vi "Number of files loaded.vi"(0 "APG Config":T1, 5 "IPF temp Folder":path, 11 "error in (no error)":errorcluster) -> (15 "error out":errorcluster)   [LabVIEW 2013, in "Manipulate IPF.lvlib"]
uses:
  Manipulate IPF.lvlib
  Settings/type_def/APG Config.ctl
  <userlib>/_OpenG.lib/file/file.llb/File Exists - Scalar__ogtk.vi
  <userlib>/_OpenG.lib/file/file.llb/Valid Path - Traditional__ogtk.vi
  a3Di APG.lvlib
  Settings/APG_settings.lvlib
panel:
  out "# of file loaded":string
  # "IPF Files Loaded"
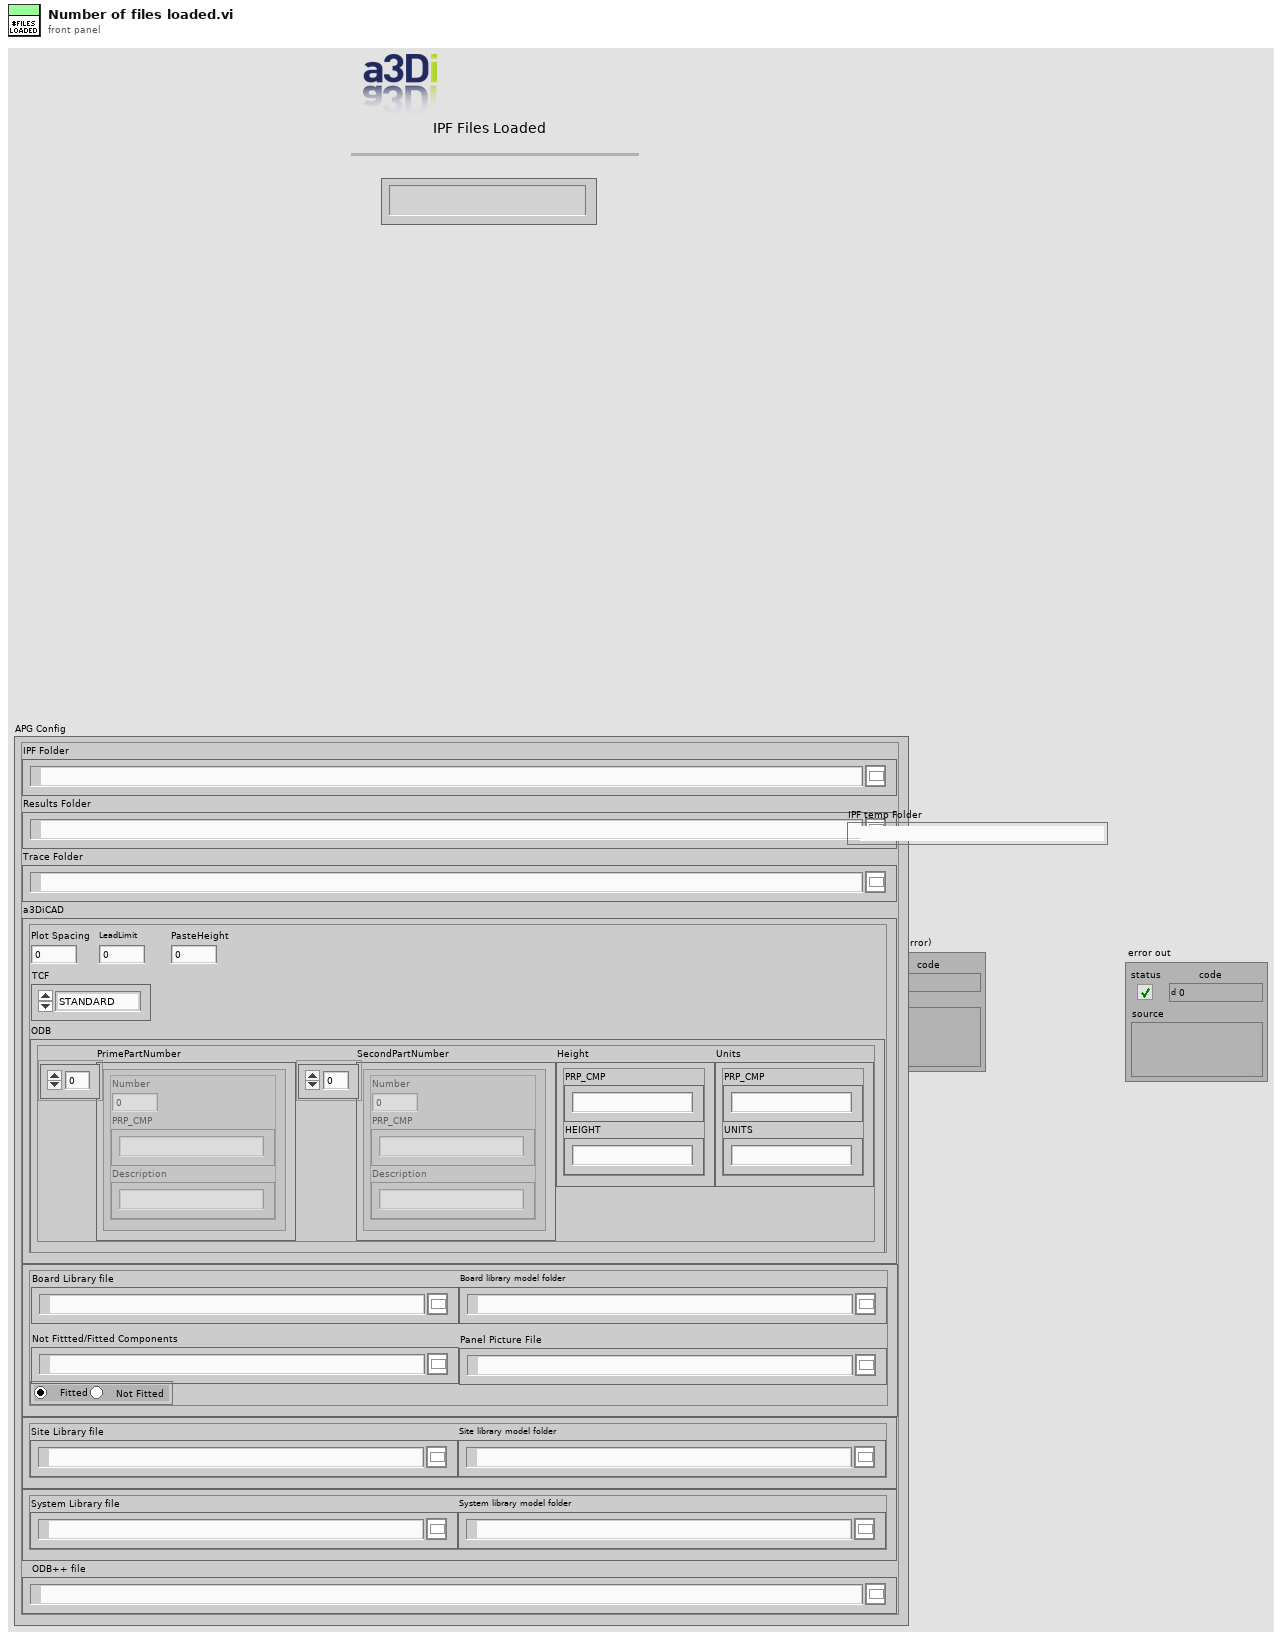
[diagram p1: front panel]
types:
  T1 = typedef "APG_settings.lvlib/APG Config.ctl" = cluster{"IPF Folder":path, "Results Folder":path, "Trace Folder":path, "a3DiCAD":cluster{"Plot Spacing":dbl, "TCF":enum16{"STANDARD", "PASTE", "LEAD"}, "LeadLimit":u32, "a3DiCADDebug":bool, "ODB":cluster{"PrimePartNumber":cluster{"Number":u32, "PRP_CMP":string, "Description":string}[], "SecondPartNumber":cluster{"Number":u32, "PRP_CMP":string, "Description":string}[], "Height":cluster{"PRP_CMP":string, "HEIGHT":string}, "Units":cluster{"PRP_CMP":string, "UNITS":string}}, "PasteHeight":dbl}, "a3DiCADcfg":path, "Board Library":cluster{"Board Library file":path, "Board library model folder":path, "Not Fittted/Fitted Components":path, "Panel Picture File":path, "Components":enum32{"Fitted", "Not Fitted "}}, "Site Library":cluster{"Site Library file":path, "Site library model folder":path}, "System Library":cluster{"System Library file":path, "System library model folder":path}, "ODB++ file":path}
  T2 = enum32{"Invalid", "Standard", "Closed", "Hidden", "Minimized", "Maximized"}
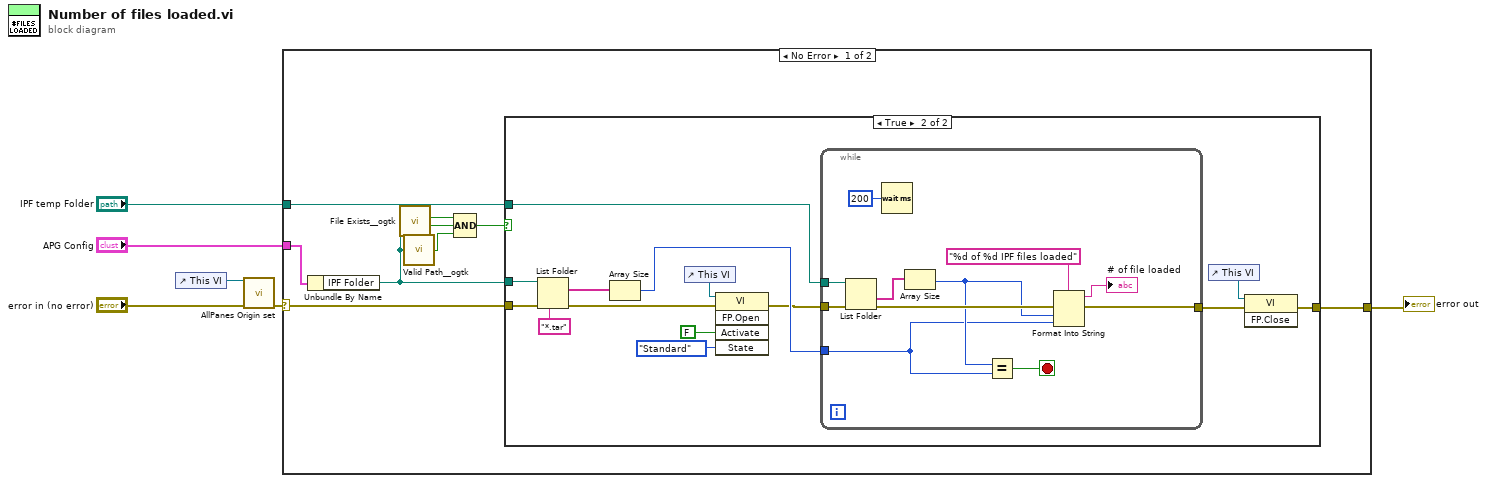
[diagram p0: block diagram]
diagram:
  n1 = control-ref of="This VI"() -> (w6:refnum<vi>)
  n2 = call "AllPanes Origin set.vi"("VI ref in"=w6, "error in"="error in (no error)") -> ("error out"=w4:errorcluster)  [unwired: 12 in, 1 out]
  n3 = case shown="No Error" w4 {
    selector: w4 -> [w13 w42]
    tunnel: "APG Config" -> [w15 _]
    tunnel: "IPF temp Folder" -> [w14 _]
    tunnel: [w12 w42] -> w1
    frame No Error {
      n4 = Unbundle By Name(w15) -> ("IPF Folder"=w11:path)
      n5 = call-poly <userlib>:"File Exists__ogtk.vi"("file path"=w11) -> ("is directory"=w10:bool, "exists"=w9:bool)  [unwired: 6 in]
      n6 = call-poly <userlib>:"Valid Path__ogtk.vi"("path"=w11) -> ("valid"=w8:bool)
      n7 = Compound Arithmetic op=AND(w10, w9, w8) -> (w7:bool)
      n8 = case shown="True" w7 {
        tunnel: w11 -> [_ w28]
        tunnel: w14 -> [_ w27]
        tunnel: w13 -> [w16 w21]
        tunnel: [w16 w17] -> w12
        frame False {
        }
        frame True {
          n9 = List Folder(path=w28, pattern="*.tar", error in=w21) -> (filenames=w29:string[], error out=w23:errorcluster)  [unwired: 1 in, 2 out]
          n10 = Array Size(array=w29) -> (size(s)=w30:i32)
          n11 = control-ref of="This VI"() -> (w24:refnum<vi>)
          n12 = invoke class="VI" method="FP.Open"(reference=w24, error in=w23, "Activate"=FALSE ("Activate?"), "State"=T2."Standard") -> (error out=w22:errorcluster)  [unwired: 1 in, 4 out]
          n13 = while {
            tunnel: w30 -> [w31]
            tunnel: w27 -> [w39]
            tunnel: w22 -> [w37]
            tunnel: [w35] -> w18
            stop <- w38 stop-if-true
            n14 = List Folder(path=w39, error in=w37) -> (folder names=w40:string[], error out=w36:errorcluster)  [unwired: 2 in, 2 out]
            n15 = Wait (ms)(milliseconds to wait=u32 200) -> ()  [unwired: 1 out]
            n16 = Array Size(array=w40) -> (size(s)=w32:i32)
            n17 = Equal?(x=w32, y=w31) -> (x = y?=w38:bool)
            n18 = Format Into String(format string="%d of %d IPF files loaded", error in=w36, w32, w31) -> (resulting string=→"# of file loaded":string, error out=w35:errorcluster)  [unwired: 1 in]
          }
          n19 = control-ref of="This VI"() -> (w19:refnum<vi>)
          n20 = invoke class="VI" method="FP.Close"(reference=w19, error in=w18) -> (error out=w17:errorcluster)  [unwired: 1 in, 2 out]
        }
      }
    }
    frame Error {
    }
  }
  "error out" <- w1
